vi "FiberSpectrograph_monitorCommand_exitControl.vi"(8 "error in (no error)":errorcluster, 11 "command_exitControl_Ctl":T1) -> (0 "error out":errorcluster, 2 "function return":i32, 3 "command_exitControl_Ctl out":T1)   [LabVIEW 2016, in "SALLV_FiberSpectrograph.lvlib"]
doc: "int FiberSpectrograph_shm_monitorCommand_exitControlLV(FiberSpectrograph_command_exitControlLV *command_exitControl_Ctl );"
uses:
  SALLV_FiberSpectrograph.lvlib
  DataTypes/command_exitControl.ctl
  SALLV_FiberSpectrograph.so
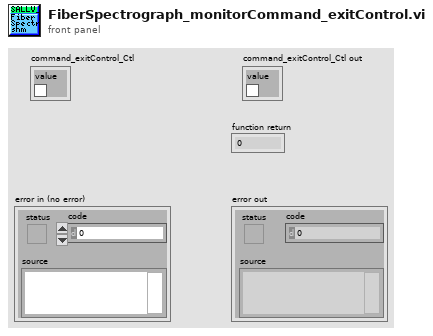
[diagram p1: front panel]
types:
  T1 = typedef "SALLV_FiberSpectrograph.lvlib/command_exitControl.ctl" = cluster{"value":bool}
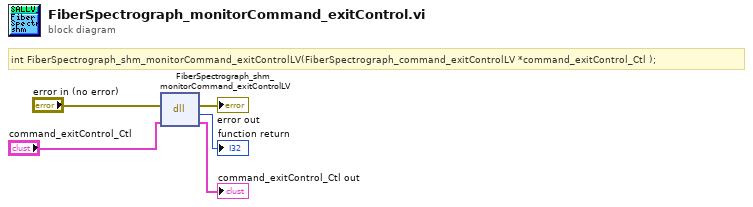
[diagram p0: block diagram]
diagram:
  # "int FiberSpectrograph_shm_monitorCommand_exitControlLV(FiberSpectrograph_command_exitControlLV *command_exitControl_Ctl );"
  n1 = dll-call lib="home/harini/tcs/temp/SALLV_FiberSpectrograph.*" fn="FiberSpectrograph_shm_monitorCommand_exitControlLV"(error in="error in (no error)", "command_exitControl_Ctl"="command_exitControl_Ctl") -> (error out=→"error out":errorcluster, →"function return":i32, "command_exitControl_Ctl"=→"command_exitControl_Ctl out":T1)  [unwired: 2 in, 1 out]
